vi "SGUI Register Controls Groups.vi"(6 "error in":errorcluster, 8 "control groups":T1(array[cluster]), 9 "groups names":string, 10 "register mode (overwrite)":T2=enum."Overwrite") -> (7 "error out":errorcluster)   [LabVIEW 2013, in "varilib.lvlib"]
doc: "This VI registers groups of controls for group control functions of SGUI lib. List of references is assigned together with name strings (multiline string, one line per group). Multiple groups are registered by single call. The primary use is for these functions is easy enabling/disabling of whole groups of controls by single command without listing them every time.\nI.e. for instance one group is stop button called 'busy', another group are buttons used for setup and start of some measurements called 'ready'. Later anywhere in the application the enable states of the controls can be changed by calling group function with 'busy' or 'ready' parameter. Number of groups is not limited. \n\nWhen sub-panel is displayed this VI can be called again to register new control groups. It can either overwrite originals or add new ones to stack. When the sub-panel is closed, thi VI may be called with 'release' parameter to remove last registered groups.\n\nWhen called for the first time in the main VI is must be called with default 'overwrite' parameter in order to get rid of residue of data in the global variable of the SGUI lib!\n\nThis VI ignores input error and will not generate error."
uses:
  varilib.lvlib
  SGUI Assign References Mode.ctl
  SGUI Global Var.vi
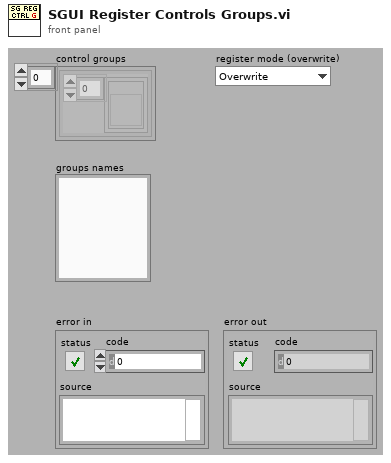
[diagram p1: front panel]
types:
  T1 = cluster{"control references (empty)":refnum<vi>[]}[]
  T2 = typedef "varilib.lvlib/SGUI Assign References Mode.ctl" = enum16{"Add to stack", "Overwrite", "Release last"}
  T3 = cluster{string[], cluster{"control references (empty)":refnum<vi>[]}[]}
  T4 = cluster{"group names":string[], "controls per goups":cluster{"control references (empty)":refnum<vi>[]}[]}[]
  T5 = cluster{string[], cluster{"control references (empty)":refnum<vi>[]}[]}[]
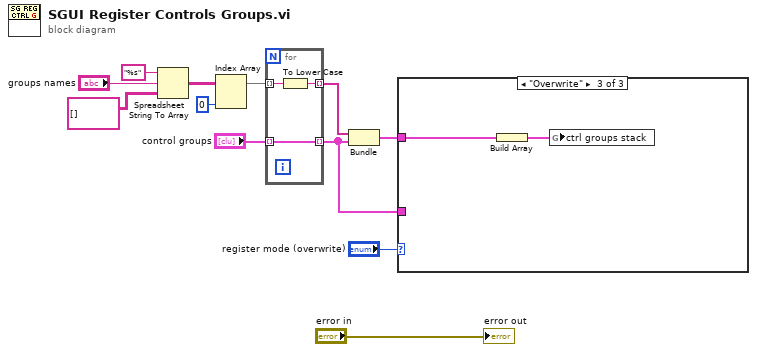
[diagram p0: block diagram]
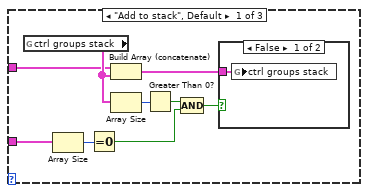
[diagram p2: hidden frame]
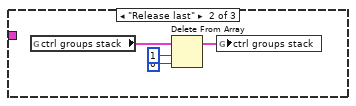
[diagram p4: hidden frame]
diagram:
  n1 = Spreadsheet String To Array(format string="%s", spreadsheet string="groups names", array type (2D Dbl)=string[][] []) -> (array=w6:string[][])  [unwired: 1 in]
  n2 = Index Array(array=w6, index (col)=0 ("disabled index (col)")) -> (element=w2:string[])  [unwired: 1 in]
  n3 = for {
    tunnel: "control groups" -> [w14] mode=indexing
    tunnel: w2 -> [w15] mode=indexing
    tunnel: [w13] -> w5 mode=indexing
    tunnel: [w14] -> w3 mode=indexing
    n4 = To Lower Case(string=w15) -> (all lower case string=w13:string)
  }
  n5 = Bundle(w5, w3) -> (w4:T3)  [unwired: 1 in]
  n6 = case shown="\"Overwrite\"" "register mode (overwrite)" {
    tunnel: w4 -> [w17 _ w31]
    tunnel: w3 -> [w16 _ _]
    frame "Add to stack", Default {
      n7 = global read "SGUI Global Var.vi" "ctrl groups stack"() -> (w20:T4)
      n8 = Array Size(array=w16) -> (size(s)=w18:i32)
      n9 = Equal To 0?(x=w18) -> (x = 0?=w22:bool)
      n10 = Build Array (concatenate)(w17, w20) -> (w19:T4)
      n11 = Array Size(array=w20) -> (size(s)=w24:i32)
      n12 = Greater Than 0?(x=w24) -> (x > 0?=w23:bool)
      n13 = Compound Arithmetic op=AND(w23, w22) -> (w21:bool)
      n14 = case shown="False" w21 {
        tunnel: w19 -> [w25 _]
        frame False {
          n15 = global write "SGUI Global Var.vi" "ctrl groups stack"(w25) -> ()
        }
        frame True {
        }
      }
    }
    frame "Release last" {
      n16 = global read "SGUI Global Var.vi" "ctrl groups stack"() -> (w29:T4)
      n17 = Delete From Array(array=w29, length=1, index=0) -> (array with subset deleted=w26:T4)  [unwired: 1 out]
      n18 = global write "SGUI Global Var.vi" "ctrl groups stack"(w26) -> ()
    }
    frame "Overwrite" {
      n19 = Build Array(w31) -> (w30:T5)
      n20 = global write "SGUI Global Var.vi" "ctrl groups stack"(w30) -> ()
    }
  }
  "error out" <- "error in"
